vi "Untitled 1.vi"() -> ()   [LabVIEW 2016]
uses:
  EDSDK131020CD(13.10.20)/EDSDK131020CD(13.10.20)/Windows/EDSDK_64/Dll/EDSDK.dll
panel:
  out "return type 3":i32
  out "return type 2":i32
  out "return type":i32
  out "Info":T1
  out "outDeviceInfo":T2
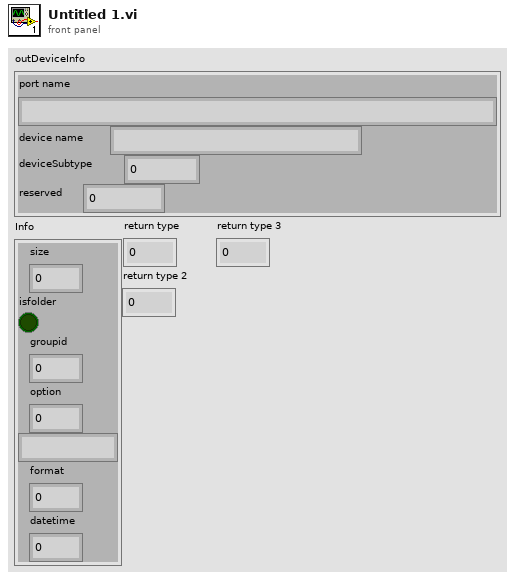
[diagram p1: front panel]
types:
  T1 = cluster{"size":u64, "isfolder":bool, "groupid":u32, "option":u32, string, "format":u32, "datetime":u32}
  T2 = cluster{"port name":string, "device name":string, "deviceSubtype":u32, "reserved":u32}
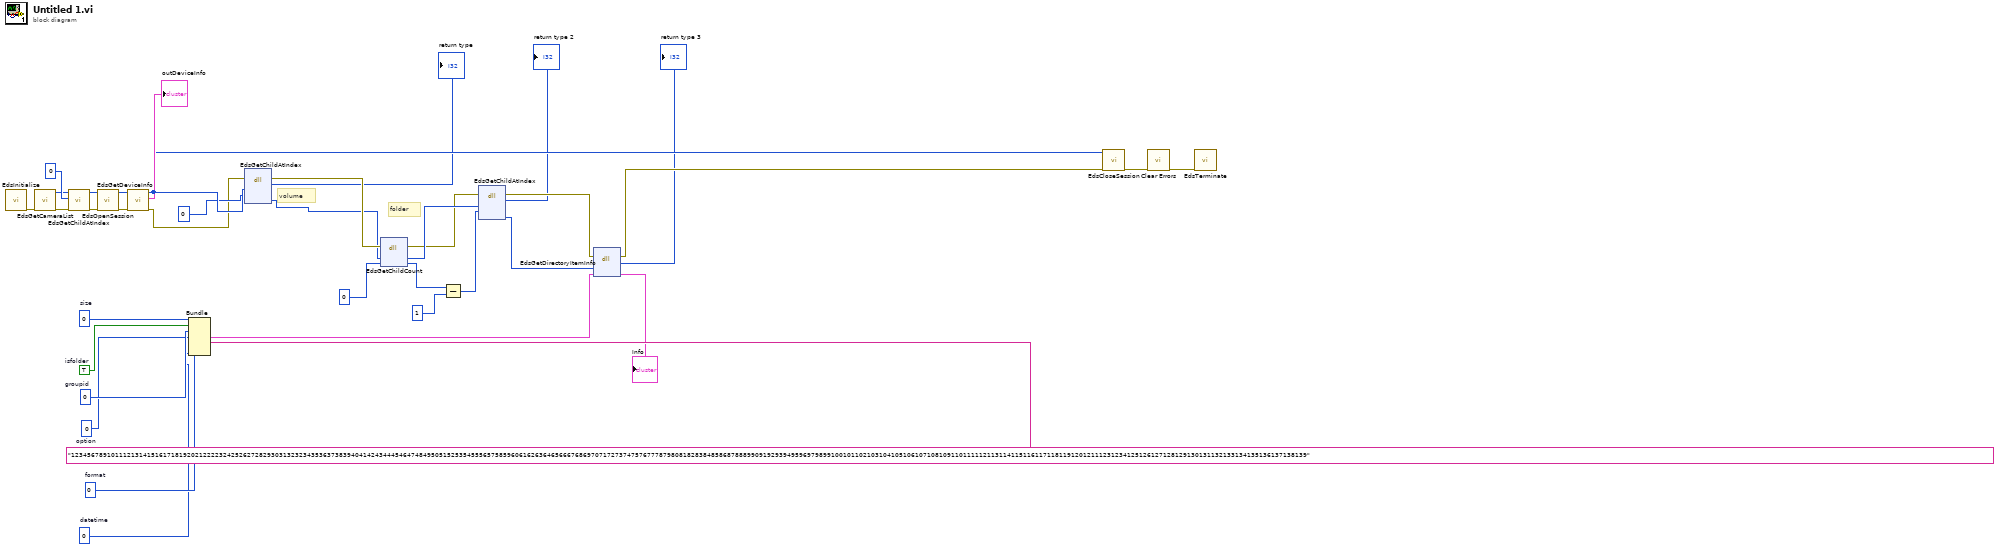
[diagram p0: block diagram]
diagram:
  w17 = u32 0  # datetime
  w18 = u32 0  # format
  w20 = u32 0  # option
  w21 = u32 0  # groupid
  w22 = TRUE  # isfolder
  w23 = u64 0  # size
  # "folder"
  # "volume"
  n1 = call "EdsInitialize.vi"() -> ("error out"=w37:errorcluster)  [unwired: 11 in]
  n2 = call "EdsGetCameraList.vi"("error in"=w37) -> ("error out"=w36:errorcluster, "outCameraListRef"=w29:u32)  [unwired: 9 in]
  n3 = call "EdsGetChildAtIndex.vi"("error in"=w36, "index"=u32 0, "inRef"=w29) -> ("error out"=w35:errorcluster, "outRef"=w33:u32)  [unwired: 7 in]
  n4 = call "EdsOpenSession.vi"("error in"=w35, "inCameraRef"=w33) -> ("error out"=w31:errorcluster, "inCameraRef dup"=w32:u32)  [unwired: 8 in]
  n5 = call "EdsGetDeviceInfo.vi"("error in"=w31, "inCameraRef"=w32) -> ("error out"=w12:errorcluster, "outDeviceInfo"=→"outDeviceInfo":T2, "inCameraRef dup"=w14:u32)  [unwired: 7 in]
  n6 = Bundle("size"=w23, "isfolder"=w22, "groupid"=w21, "option"=w20, "123456789101112131415161718192021222232425262728293031323234353637383940414243444546474849505152535455565758596061626364656667686970717273747576777879808182838485868788899091929394959697989910010110210310410510610710810911011111211311411511611711811912012111231234125126127128129130131132133134135136137138139", "format"=w18, "datetime"=w17) -> (w16:T1)  [unwired: 1 in]
  n7 = dll-call lib="D:/All Users/Summer2019/Camera_po_sheng/Canon/EDSDK131020CD(13.10.20)/EDSDK131020CD(13.10.20)/Windows/EDSDK_64/Dll/EDSDK.dll" fn="EdsGetChildAtIndex"(error in=w12, "ref"=w14, "index"=0) -> (error out=w11:errorcluster, "return type"=→"return type":i32, "outref"=w10:u32)  [unwired: 5 in, 1 out]
  n8 = dll-call lib="D:/All Users/Summer2019/Camera_po_sheng/Canon/EDSDK131020CD(13.10.20)/EDSDK131020CD(13.10.20)/Windows/EDSDK_64/Dll/EDSDK.dll" fn="EdsGetChildCount"(error in=w11, "ref"=w10, "childcount"=u32 0) -> (error out=w5:errorcluster, "ref"=w7:u32, "childcount"=w24:u32)  [unwired: 3 in, 1 out]
  n9 = Subtract(x=w24, y=u32 1) -> (x-y=w8:u32)
  n10 = dll-call lib="D:/All Users/Summer2019/Camera_po_sheng/Canon/EDSDK131020CD(13.10.20)/EDSDK131020CD(13.10.20)/Windows/EDSDK_64/Dll/EDSDK.dll" fn="EdsGetChildAtIndex"(error in=w5, "ref"=w7, "index"=w8) -> (error out=w4:errorcluster, "return type"=→"return type 2":i32, "outref"=w6:u32)  [unwired: 5 in, 1 out]
  n11 = dll-call lib="D:/All Users/Summer2019/Camera_po_sheng/Canon/EDSDK131020CD(13.10.20)/EDSDK131020CD(13.10.20)/Windows/EDSDK_64/Dll/EDSDK.dll" fn="EdsGetDirectoryItemInfo"(error in=w4, "ref"=w6, "Info"=w16) -> (error out=w2:errorcluster, "return type"=→"return type 3":i32, "Info"=→"Info":T1)  [unwired: 3 in, 1 out]
  n12 = call "EdsCloseSession.vi"("error in"=w2, "inCameraRef"=w14) -> ("error out"=w28:errorcluster)  [unwired: 8 in, 1 out]
  n13 = call <vilib>:"Clear Errors.vi"("error in (no error)"=w28) -> ("error out"=w27:errorcluster)  [unwired: 5 in, 1 out]
  n14 = call "EdsTerminate.vi"("error in"=w27) -> ()  [unwired: 10 in, 1 out]
